vi "2_Hot_Films_Prep.vi"() -> (5 "Plug in titles":string[](array[string]), 7 "Plug in values":string[](array[string]))   [LabVIEW 2010]
uses:
  Controls/Post_Process.ctl
  Globals/Meas_global.vi
  Globals/Plug_in_data_global.vi
  <vilib>/Analysis/3filter.llb/Butterworth Filter (DBL).vi
  <vilib>/Analysis/NI_AALBase.lvlib
panel:
  in  "Block Length":i32=2500
  out "U components":cluster{dbl[], dbl[]}[](graph)
  out "Iteration No":i32
  out "XY Graph":cluster{i32[], dbl[]}[](graph)
  in  "Approx Delay (s)":dbl=23.0 format="%.2f"
  in  "Approx period":dbl=80.0 format="%.2f"
  in  "End Chop":i32=500
  in  "Start Chop":i32=2500
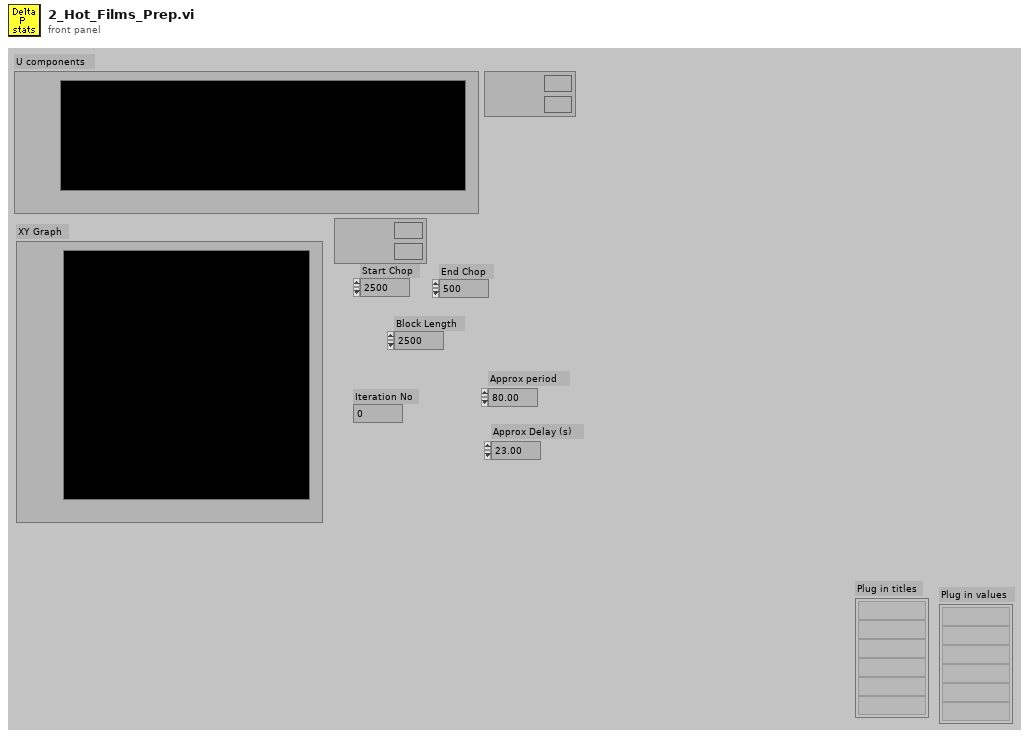
[diagram p1: front panel]
types:
  T1 = enum32{"Lowpass", "Highpass", "Bandpass", "Bandstop"}
  T2 = typedef "Post_Process.ctl" = enum16{"Take New Data", "Post Process Raw Data File"}
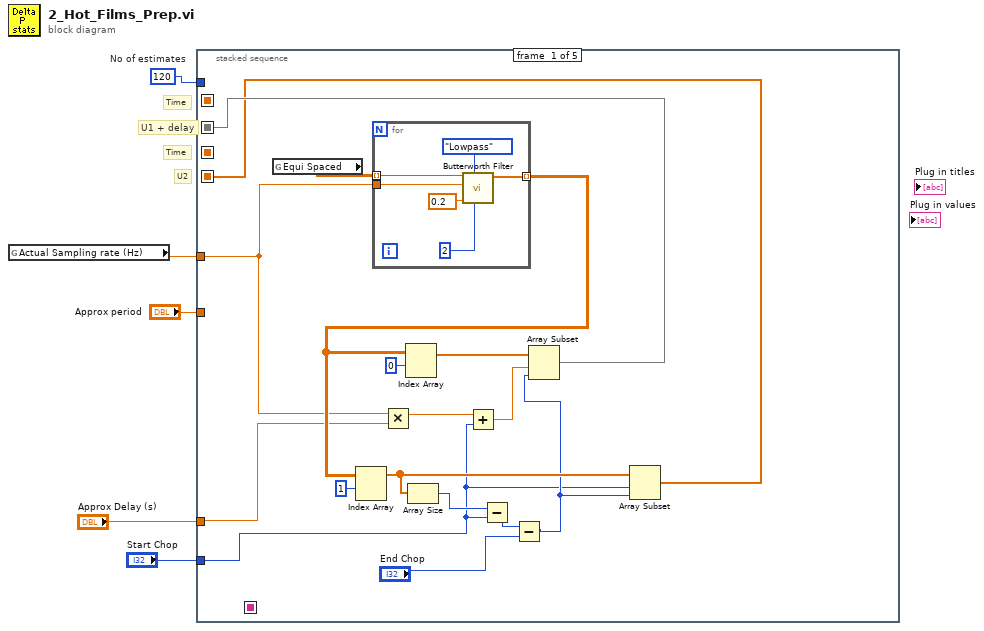
[diagram p0: block diagram]
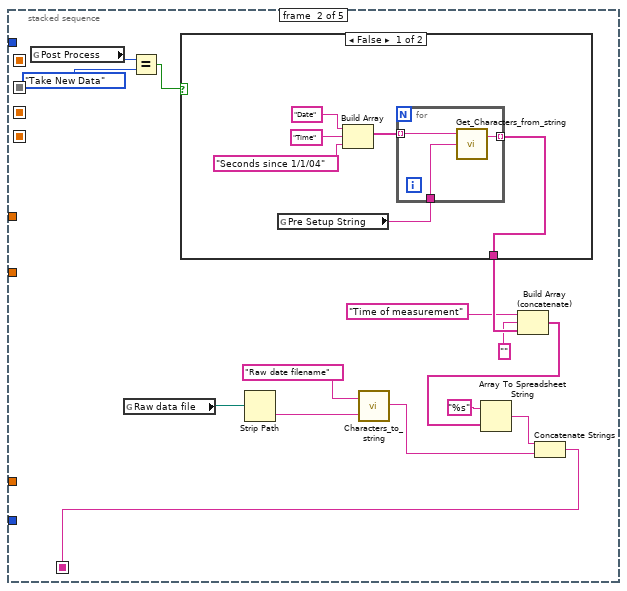
[diagram p2: hidden frame]
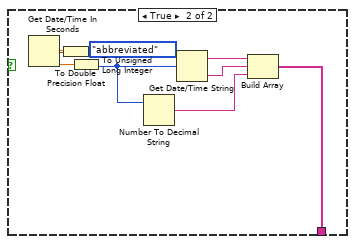
[diagram p3: hidden frame]
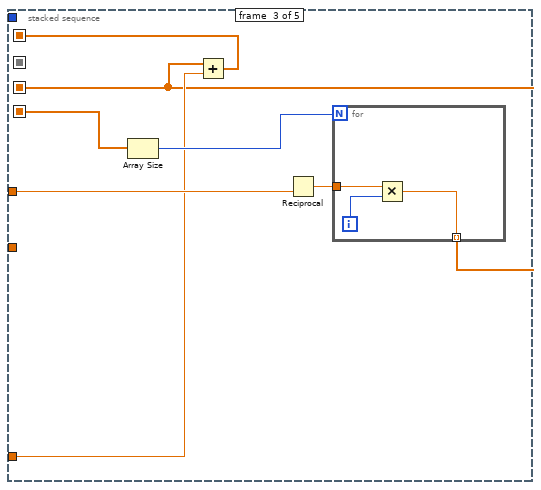
[diagram p4: hidden frame]
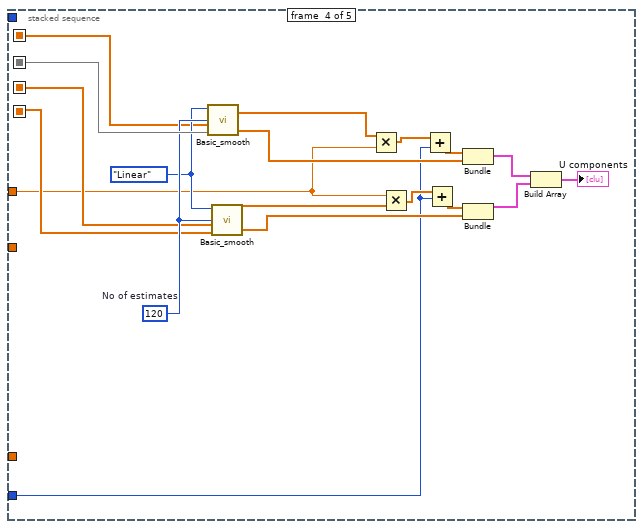
[diagram p5: hidden frame]
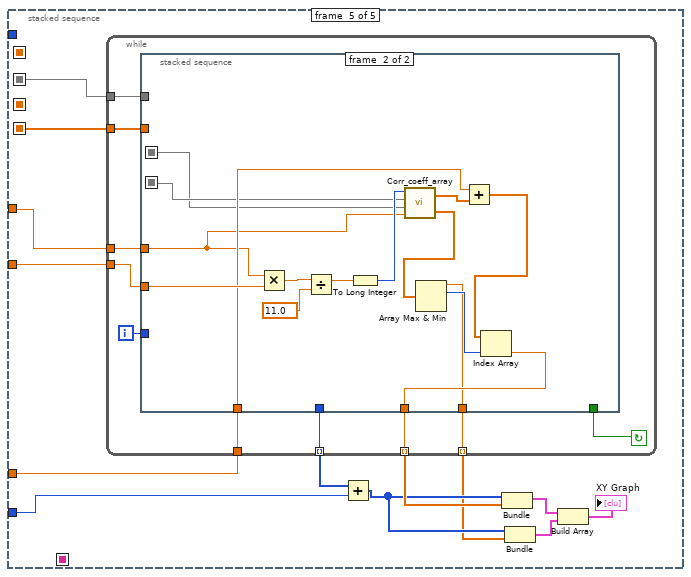
[diagram p6: hidden frame]
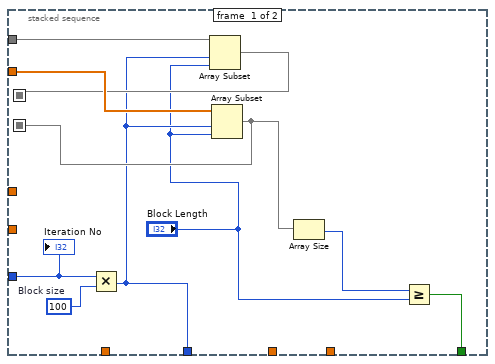
[diagram p7: hidden frame]
diagram:
  w5 = 120  # No of estimates
  # "Time"
  # "Time"
  # "U2"
  # "U1 + delay"
  n1 = global read "Meas_global.vi" "Actual Sampling rate (Hz)"() -> (w3:dbl)
  n2 = stacked-sequence {
    seq-local: [_ w35 _ _ _] -> [_ _ _ _ _]
    seq-local: [w13 _ _ _ _] -> [_ _ _ w88 w98]
    seq-local: [w12 _ _ _ _] -> [_ _ w64 w78 w97]
    seq-local: [_ _ w60 _ _] -> [_ _ _ w80 _]
    seq-local: [_ _ w61 _ _] -> [_ _ _ w79 _]
    tunnel: w3 -> [w16 _ w65 w75 w100]
    tunnel: w5 -> [_ _ _ _ _]
    tunnel: "Approx period" -> [_ _ _ _ w101]
    tunnel: "Approx Delay (s)" -> [w17 _ w62 _ w99]
    tunnel: "Start Chop" -> [w6 _ _ w72 w94]
    frame #0 {
      n3 = global read "Plug_in_data_global.vi" "Equi Spaced"() -> (w22:dbl[][])
      n4 = for {
        tunnel: [w25] -> w19 mode=indexing
        tunnel: w16 -> [w24]
        tunnel: w22 -> [w23] mode=indexing
        n5 = call-poly <vilib>:"Butterworth Filter.vi"("order"=2, "filter type"=T1."Lowpass", "low cutoff freq: fl"=0.2, "sampling freq: fs"=w24, "X"=w23) -> ("Filtered X"=w25:dbl[])  [unwired: 3 in, 1 out]
      }
      n6 = Index Array(array=w19, index (row)=1 ("Index")) -> (element=w11:dbl[])  [unwired: 1 in]
      n7 = Multiply(x=w16, y=w17) -> (x*y=w15:dbl)
      n8 = Index Array(array=w19, index (row)=0 ("Index")) -> (element=w18:dbl[])  [unwired: 1 in]
      n9 = Array Size(array=w11) -> (size(s)=w10:i32)
      n10 = Add(x=w15, y=w6) -> (x+y=w14:dbl)
      n11 = Subtract(x=w10, y=w6) -> (x-y=w9:i32)
      n12 = Subtract(x=w9, y="End Chop") -> (x-y=w7:i32)
      n13 = Array Subset(array=w18, index=w14, length=w7) -> (w13:dbl[])
      n14 = Array Subset(array=w11, index=w6, length=w7) -> (w12:dbl[])
    }
    frame #1 {
      n15 = global read "Meas_global.vi" "Post Process"() -> (w41:T2)
      n16 = global read "Meas_global.vi" "Raw data file"() -> (w30:path)
      n17 = Equal?(x=w41, y=Post_Process."Take New Data" ("Post Process")) -> (x = y?=w40:bool)
      n18 = case shown="False" w40 {
        tunnel: [w43 w53] -> w34
        frame False {
          n19 = global read "Meas_global.vi" "Pre Setup String"() -> (w44:string)
          n20 = Build Array("Date", "Time", "Seconds since 1/1/04") -> (w45:string[])
          n21 = for {
            tunnel: w45 -> [w51] mode=indexing
            tunnel: w44 -> [w50]
            tunnel: [w49] -> w43 mode=indexing
            n22 = call "Get_Characters_from_string.vi"("Input string"=w50, "Variable name"=w51) -> ("Value"=w49:string)  [unwired: 1 in, 1 out]
          }
        }
        frame True {
          n23 = Get Date/Time In Seconds() -> (seconds since 1Jan1904=w52:timestamp)
          n24 = To Double Precision Float(number=w52) -> (double precision float=w56:dbl)
          n25 = To Unsigned Long Integer(number=w56) -> (unsigned 32bit integer=w55:u32)
          n26 = Number To Decimal String(number=w55) -> (decimal integer string=w54:string)  [unwired: 1 in]
          n27 = Get Date/Time String(date format (0)=enum16{"short", "long", "abbreviated"}."abbreviated", seconds (now)=w55) -> (date string=w58:string, time string=w57:string)  [unwired: 1 in]
          n28 = Build Array(w58, w57, w54) -> (w53:string[])
        }
      }
      n29 = Strip Path(path=w30) -> (name=w29:string)  [unwired: 1 out]
      n30 = call "Characters_to_string.vi"("Characters to write"=w29, "Label for characters"="Raw date filename") -> ("Output string"=w36:string)
      n31 = Build Array (concatenate)("Time of measurement", "" ("Value"), w34) -> (w31:string[])
      n32 = Array To Spreadsheet String(array=w31, 3:"%s" ("format string")) -> (spreadsheet string=w37:string)  [unwired: 1 in]
      n33 = Concatenate Strings(w37, w36) -> (w35:string)
    }
    frame #2 {
      n34 = Array Size(array=w64) -> (size(s)=w63:i32)
      n35 = Reciprocal(x=w65) -> (1/x=w66:dbl)
      n36 = for {
        N: w63 -> [_]
        tunnel: w66 -> [w69]
        tunnel: [w67] -> w61 mode=indexing
        i -> [w68]
        n37 = Multiply(x=w69, y=w68) -> (x*y=w67:dbl)
      }
      n38 = Add(x=w61, y=w62) -> (x+y=w60:dbl[])
    }
    frame #3 {
      w86 = 120  # No of estimates
      w84 = enum16{"Linear", "Logarithmic"}."Linear" ("Smoothing")
      n39 = call "Basic_smooth.vi"("Smoothing"=w84, "X array in"=w80, "Y array in"=w88, "No of estimates output"=w86) -> ("X array Out"=w77:dbl[], "Y array Out"=w83:dbl[])  [unwired: 1 in]
      n40 = call "Basic_smooth.vi"("Smoothing"=w84, "X array in"=w79, "Y array in"=w78, "No of estimates output"=w86) -> ("X array Out"=w76:dbl[], "Y array Out"=w85:dbl[])  [unwired: 1 in]
      n41 = Multiply(x=w77, y=w75) -> (x*y=w73:dbl[])
      n42 = Multiply(x=w75, y=w76) -> (x*y=w74:dbl[])
      n43 = Add(x=w73, y=w72) -> (x+y=w71:dbl[])
      n44 = Add(x=w74, y=w72) -> (x+y=w70:dbl[])
      n45 = Bundle(w71, "Y array Out"=w83) -> (w81:cluster{dbl[], "Y array Out":dbl[]})  [unwired: 1 in]
      n46 = Bundle(w70, "Y array Out"=w85) -> (w82:cluster{dbl[], "Y array Out":dbl[]})  [unwired: 1 in]
      n47 = Build Array(w81, w82) -> (→"U components":cluster{dbl[], "Y array Out":dbl[]}[])
    }
    frame #4 {
      n48 = while {
        tunnel: [w102] -> w92 mode=indexing
        tunnel: [w103] -> w96 mode=indexing
        tunnel: [w104] -> w95 mode=indexing
        tunnel: w97 -> [w106]
        tunnel: w98 -> [w108]
        tunnel: w99 -> [w109]
        tunnel: w100 -> [w110]
        tunnel: w101 -> [w111]
        i -> [w107]
        stop <- w105 continue-if-true
        n49 = stacked-sequence {
          seq-local: [w115 _] -> [_ w127]
          seq-local: [w114 _] -> [_ w128]
          tunnel: w111 -> [_ w136]
          tunnel: w110 -> [_ w129]
          tunnel: w109 -> [_ w130]
          tunnel: w108 -> [w121 _]
          tunnel: w107 -> [w120 _]
          tunnel: w106 -> [w118 _]
          tunnel: [w116 _] -> w105
          tunnel: [w113 _] -> w104
          tunnel: [_ w123] -> w103
          tunnel: [_ w122] -> w102
          frame #0 {
            w119 = 100  # Block size
            n50 = Multiply(x=w120, y=w119) -> (x*y=w113:i32)
            n51 = Array Subset(array=w121, index=w113, length="Block Length") -> (w115:dbl[])
            n52 = Array Subset(array=w118, index=w113, length="Block Length") -> (w114:dbl[])
            n53 = Array Size(array=w114) -> (size(s)=w117:i32)
            n54 = Greater Or Equal?(x=w117, y="Block Length") -> (x >= y?=w116:bool)
            "Iteration No" <- w120
          }
          frame #1 {
            n55 = Multiply(x=w129, y=w136) -> (x*y=w134:dbl)
            n56 = Divide(x=w134, y=11.0) -> (x/y=w132:dbl)
            n57 = To Long Integer(number=w132) -> (32bit integer=w135:i32)
            n58 = call "Corr_coeff_array.vi"("Sampling frequency"=w129, "U2"=w127, "U1"=w128, "Slippage range"=w135) -> ("Correlation Coefficient"=w125:dbl[], "Time"=w131:dbl[])
            n59 = Array Max & Min(array=w125) -> (max value=w122:dbl, max index (indices)=w126:i32)  [unwired: 2 out]
            n60 = Add(x=w130, y=w131) -> (x+y=w124:dbl[])
            n61 = Index Array(array=w124, index=w126) -> (element=w123:dbl)
          }
        }
      }
      n62 = Add(x=w95, y=w94) -> (x+y=w93:i32[])
      n63 = Bundle(w93, w96) -> (w91:cluster{i32[], dbl[]})  [unwired: 1 in]
      n64 = Bundle(w93, w92) -> (w90:cluster{i32[], dbl[]})  [unwired: 1 in]
      n65 = Build Array(w91, w90) -> (→"XY Graph":cluster{i32[], dbl[]}[])
    }
  }
